vi "avg intensity plots.vi"(10 "length":i32, 11 "Intensity Graph 12":dbl[][](graph)) -> (3 "Intensity Graph 13":dbl[][](graph))   [LabVIEW 2016]
uses:
  <vilib>/Analysis/baseanly.llb/Mean (DBL).vi
  <vilib>/Analysis/NI_AALBase.lvlib
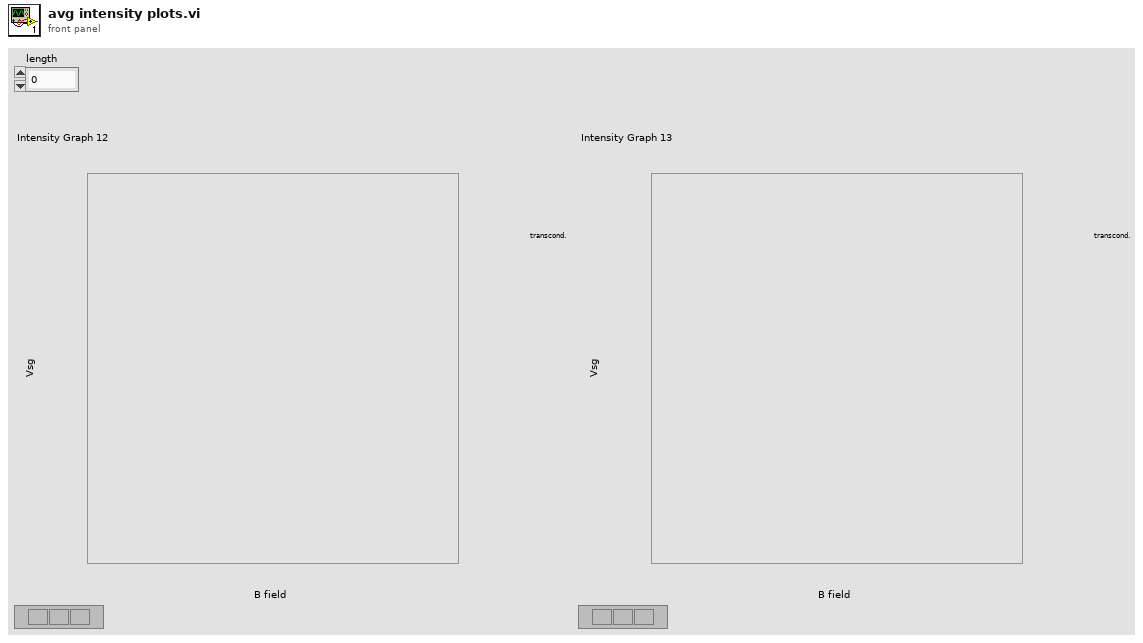
[diagram p1: front panel]
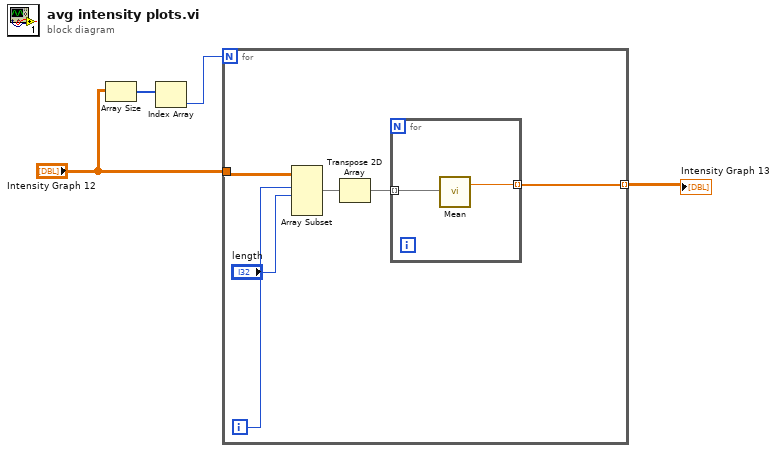
[diagram p0: block diagram]
diagram:
  n1 = Array Size(array="Intensity Graph 12") -> (size(s)=w3:i32[])
  n2 = Index Array(array=w3) -> (element=w2:i32)  [unwired: 1 in]
  n3 = for {
    N: w2 -> [_]
    tunnel: "Intensity Graph 12" -> [w10]
    tunnel: [w5] -> w1 mode=indexing
    i -> [w9]
    n4 = Array Subset(array=w10, index (row)=w9, length (row)="length") -> (w7:dbl[][])  [unwired: 2 in]
    n5 = Transpose 2D Array(2D array=w7) -> (transposed array=w6:dbl[][])
    n6 = for {
      tunnel: w6 -> [w12] mode=indexing
      tunnel: [w11] -> w5 mode=indexing
      n7 = call-poly <vilib>:"Mean.vi"("X"=w12) -> ("mean"=w11:dbl)  [unwired: 1 out]
    }
  }
  "Intensity Graph 13" <- w1
